vi "Main.vi"   [LabVIEW 2020, in "Summer of LabVIEW.lvlib" / "SOL-Server.lvclass"]
uses:
  SOL-Server.lvclass
panel:
  # "Summer of LabVIEW\nMain"
types:
  T1 = enum32{"invalid app kind", "Development System", "Run Time System", "Student Edition", "Embedded LabVIEW", "Evaluation", "Custom"}
  T2 = enum32{"Invalid", "Standard", "Closed", "Hidden", "Minimized", "Maximized"}
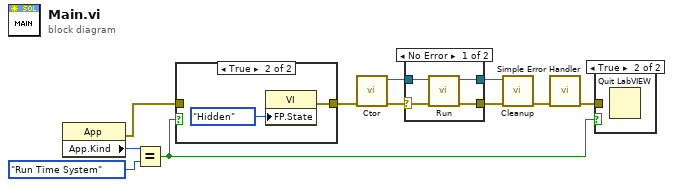
[diagram p0: block diagram]
diagram:
  n1 = property class="App"() -> (error out=w1:errorcluster, "App.Kind"=w11:T1)  [unwired: 2 in, 1 out]
  n2 = Equal?(x=w11, y=T1."Run Time System" ("Application:Kind")) -> (x = y?=w9:bool)
  n3 = case shown="True" w9 {
    tunnel: [w12 w13] -> w7
    tunnel: w1 -> [w12 _]
    frame False {
    }
    frame True {
      n4 = property class="VI"("FP.State"=T2."Hidden" ("Front Panel Window:State")) -> (error out=w13:errorcluster)  [unwired: 2 in, 1 out]
    }
  }
  n5 = call "Ctor.vi"("error in (no error)"=w7) -> ("error out"=w6:errorcluster, "SOL-Server out"=w5:refnum<class "SOL-Server.lvclass">)  [unwired: 9 in]
  n6 = case shown="No Error" w6 {
    selector: w6 -> [w17 w19]
    tunnel: w5 -> [w18 w20]
    tunnel: [w16 w20] -> w4
    tunnel: [w15 w19] -> w3
    frame No Error {
      n7 = call "Run.vi"("error in (no error)"=w17, "SOL-Server in"=w18) -> ("error out"=w15:errorcluster, "SOL-Server out"=w16:refnum<class "SOL-Server.lvclass">)  [unwired: 8 in]
    }
    frame Error {
    }
  }
  n8 = call "Cleanup.vi"("error in (no error)"=w3, "SOL-Server in"=w4) -> ("error out"=w2:errorcluster)  [unwired: 9 in]
  n9 = call <vilib>:"Simple Error Handler.vi"("error in (no error)"=w2) -> ("error out"=w8:errorcluster)  [unwired: 4 in, 4 out]
  n10 = case shown="True" w9 {
    tunnel: w8 -> [_ _]
    frame False {
    }
    frame True {
      n11 = Quit LabVIEW() -> ()  [unwired: 1 in]
    }
  }
